vi "Byte Count to U32 Transfers.vi"(11 "bytes to transfer":u32) -> (3 "U32 transfers":u32, 5 "U8 transfers":u32)   [LabVIEW 2016, in "GE 5565PIORC.lvclass"]
uses:
  GE 5565PIORC.lvclass
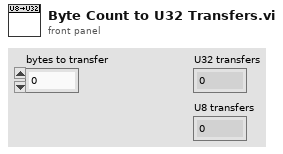
[diagram p1: front panel]
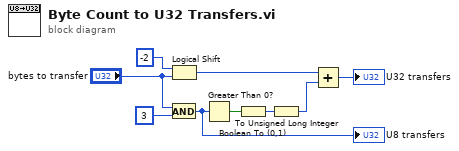
[diagram p0: block diagram]
diagram:
  n1 = Logical Shift(y=i16 -2, x="bytes to transfer") -> (x << y=w5:u32)
  n2 = And(x="bytes to transfer", y=u32 3) -> (x .and. y?=w6:u32)
  "U8 transfers" <- w6
  n3 = Greater Than 0?(x=w6) -> (x > 0?=w4:bool)
  n4 = Boolean To (0,1)(Boolean=w4) -> (0, 1=w3:i16)
  n5 = To Unsigned Long Integer(number=w3) -> (unsigned 32bit integer=w2:u32)
  n6 = Add(x=w5, y=w2) -> (x+y=→"U32 transfers":u32)
